vi "create run list.vi"(7 "Group Stanards":string[][](array[string]), 8 "error in (no error)":errorcluster, 9 "Group Unknowns":string[][](array[string]), 10 "Paged groups":string[][][](array[string])=[[["", "", "", "", "", "", ""], ["", "", "", "", "", "", ""], ["", "", "", "", "", "", ""], ["", "", "", "", "", "", ""], ["", "", "", "", "", "", ""], ["", "", "", "", "", "", ""], ["", "", "", "", "", "", ""], ["", "", "", "", "", "", ""], ["", "", "", "", "", "", ""], ["", "", "", "", "", "", ""], ["", "", "", "", "", "", ""], ["", "", "", "", "", "", ""], ["", "", "", "", "", "", ""], ["", "", "", "", "", "", ""]], [["1", "113250", "Owen", "JDP1", "u", "1000", "1"], ["2", "113251", "Owen", "JDP2", "u", "1000", "1"], ["3", "113252", "Owen", "JDP3", "u", "1000", "1"], ["4", "113253", "Owen", "JDP4", "u", "1000", "1"], ["5", "113254", "Owen", "JB1", "u", "1000", "1"], ["6", "113255", "Owen", "JB2", "u", "1000", "1"], ["7", "113256", "Owen", "JB3", "u", "1000", "1"], ["8", "113257", "Owen", "JAC1", "u", "1000", "1"], ["9", "113258", "Owen", "BLK 4", "u", "1000", "1"], ["10", "113259", "Arboleya", "E1", "u", "1000", "1"], ["51", "110511", "Caffee", "KN std Be 0162", "u", "533", "1"], ["52", "110824", "Chmiel", "Blank", "b", "5", "1"], ["55", "96431", "Caffee", "Be-01-5-3 standard", "s", "6320", "1"], ["56", "96432", "Caffee", "Be-01-5-3 standard", "s", "6320", "1"]], [["11", "113260", "Arboleya", "E3", "u", "1000", "2"], ["12", "113261", "Arboleya", "E4", "u", "1000", "2"], ["13", "113262", "Arboleya", "E5", "u", "1000", "2"], ["14", "113263", "Arboleya", "E6", "u", "1000", "2"], ["15", "113264", "Arboleya", "E7", "u", "1000", "2"], ["16", "113265", "Arboleya", "E8", "u", "1000", "2"], ["17", "113266", "Arboleya", "E9", "u", "1000", "2"], ["18", "113267", "Arboleya", "MAR7", "u", "1000", "2"], ["19", "113268", "Arboleya", "BLK7", "u", "1000", "2"], ["20", "113269", "Marshall", "CR101", "u", "1000", "2"], ["57", "96433", "Caffee", "Be-01-5-3 standard", "s", "6320", "2"], ["58", "96434", "Caffee", "Be-01-5-3 standard", "s", "6320", "2"], ["", "", "", "", "", "", ""], ["", "", "", "", "", "", ""]], [["21", "113270", "Marshall", "CR102", "u", "1000", "3"], ["22", "113271", "Marshall", "CR103", "u", "1000", "3"], ["23", "113272", "Marshall", "CR104", "u", "1000", "3"], ["24", "113273", "Marshall", "CR106", "u", "1000", "3"], ["25", "113274", "Marshall", "CR107", "u", "1000", "3"], ["26", "113275", "Marshall", "CR109", "u", "1000", "3"], ["27", "113276", "Marshall", "CR110", "u", "1000", "3"], ["28", "113277", "Marshall", "CR111", "u", "1000", "3"], ["29", "113278", "Marshall", "CR116", "u", "1000", "3"], ["30", "113279", "Marshall", "BLK1", "u", "1000", "3"], ["31", "113280", "Marshall", "CR113", "u", "1000", "3"], ["59", "96435", "Caffee", "Be-01-5-3 standard", "s", "6320", "3"], ["60", "96436", "Caffee", "Be-01-5-3 standard", "s", "6320", "3"], ["", "", "", "", "", "", ""]], [["32", "113281", "Marshall", "CR121", "u", "1000", "4"], ["33", "113282", "Marshall", "CR122", "u", "1000", "4"], ["34", "113283", "Belmont", "W10Vi23I", "u", "1000", "4"], ["35", "113284", "Belmont", "S10X07B", "u", "1000", "4"], ["36", "113285", "Belmont", "S10X08A", "u", "1000", "4"], ["37", "113286", "Belmont", "S10X08B", "u", "1000", "4"], ["38", "113287", "Belmont", "S10X08C", "u", "1000", "4"], ["39", "113288", "Belmont", "S10X08D", "u", "1000", "4"], ["40", "113289", "Belmont", "S10X08E", "u", "1000", "4"], ["41", "113290", "Belmont", "S10X08F", "u", "1000", "4"], ["61", "96437", "Caffee", "Be-01-5-3 standard", "s", "6320", "4"], ["62", "96438", "Caffee", "Be-01-5-3 standard", "s", "6320", "4"], ["", "", "", "", "", "", ""], ["", "", "", "", "", "", ""]], [["42", "113291", "Belmont", "S10X08G", "u", "1000", "5"], ["43", "113292", "Belmont", "Cblk-2560-7", "u", "1000", "5"], ["44", "113293", "Belmont", "S10X08H", "u", "1000", "5"], ["45", "113294", "Belmont", "S10X08I", "u", "1000", "5"], ["46", "113295", "Belmont", "S10X08J", "u", "1000", "5"], ["47", "113296", "Belmont", "S10X08K", "u", "1000", "5"], ["48", "113297", "Belmont", "S10X08L", "u", "1000", "5"], ["49", "113298", "Belmont", "S10X09A", "u", "1000", "5"], ["50", "113299", "Belmont", "S10X09B", "u", "1000", "5"], ["54", "96430", "Caffee", "Be-01-5-3 standard", "s", "6320", "5"], ["63", "96439", "Caffee", "Be-01-5-3 standard", "s", "6320", "5"], ["", "", "", "", "", "", ""], ["", "", "", "", "", "", ""], ["", "", "", "", "", "", ""]], [["", "", "", "", "", "", ""], ["", "", "", "", "", "", ""], ["", "", "", "", "", "", ""], ["", "", "", "", "", "", ""], ["", "", "", "", "", "", ""], ["", "", "", "", "", "", ""], ["", "", "", "", "", "", ""], ["", "", "", "", "", "", ""], ["", "", "", "", "", "", ""], ["", "", "", "", "", "", ""], ["", "", "", "", "", "", ""], ["", "", "", "", "", "", ""], ["", "", "", "", "", "", ""], ["", "", "", "", "", "", ""]], [["", "", "", "", "", "", ""], ["", "", "", "", "", "", ""], ["", "", "", "", "", "", ""], ["", "", "", "", "", "", ""], ["", "", "", "", "", "", ""], ["", "", "", "", "", "", ""], ["", "", "", "", "", "", ""], ["", "", "", "", "", "", ""], ["", "", "", "", "", "", ""], ["", "", "", "", "", "", ""], ["", "", "", "", "", "", ""], ["", "", "", "", "", "", ""], ["", "", "", "", "", "", ""], ["", "", "", "", "", "", ""]]], 11 "number of samples between standards":i32=4 min=1 max=50) -> (0 "error out":errorcluster, 3 "Group run list":string[][](array[string]))   [LabVIEW 2016]
doc: "This vi takes the standard and unknown list data for a group and parses it into a run order"
panel:
  in  "number of times measured":i32=2
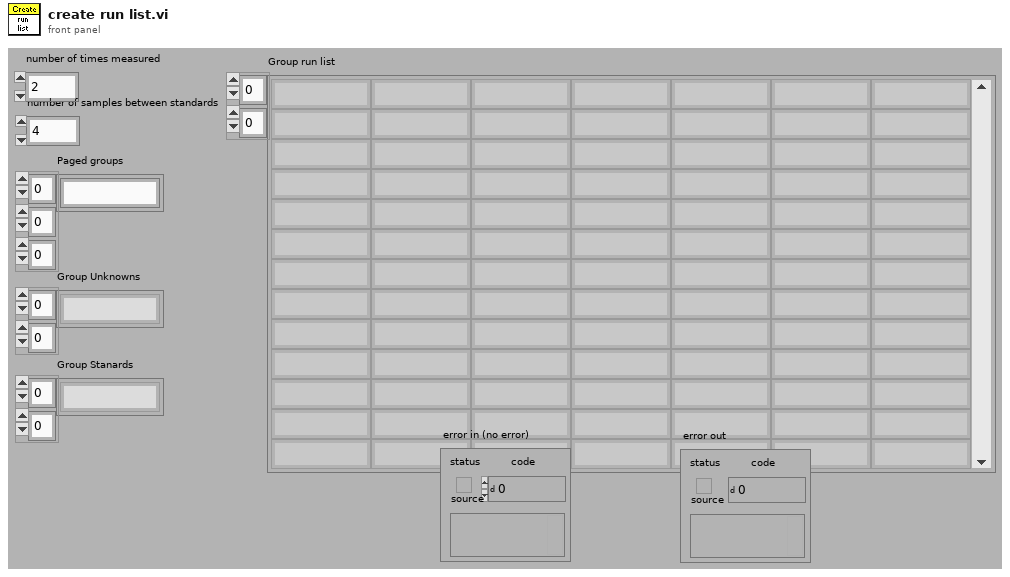
[diagram p1: front panel]
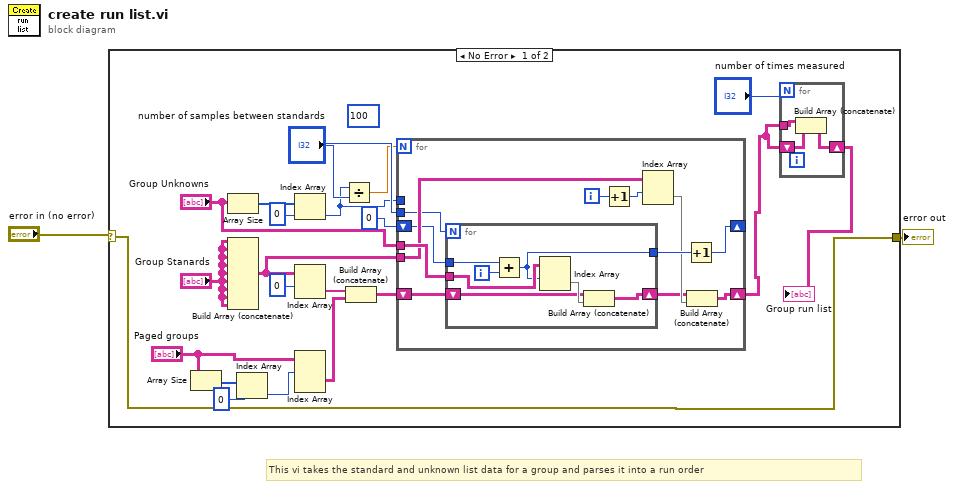
[diagram p0: block diagram]
diagram:
  # "This vi takes the standard and unknown list data for a group and parses it into a run order"
  n1 = case shown="No Error" "error in (no error)" {
    selector: "error in (no error)" -> [w11 w46]
    tunnel: [w11 w46] -> w1
    frame No Error {
      (unwired) 100
      n2 = Array Size(array="Paged groups") -> (size(s)=w9:i32[])
      n3 = Array Size(array="Group Unknowns") -> (size(s)=w13:i32[])
      n4 = Build Array (concatenate)("Group Stanards", "Group Stanards", "Group Stanards", "Group Stanards", "Group Stanards", "Group Stanards", "Group Stanards", "Group Stanards", "Group Stanards") -> (w18:string[][])
      n5 = Index Array(array=w9, index=0) -> (element=w7:i32)
      n6 = Index Array(array=w13, index=0) -> (element=w16:i32)
      n7 = Index Array(array=w18, index (row)=0) -> (element=w20:string[])  [unwired: 1 in]
      n8 = Index Array(array="Paged groups", index (dim 0)=w7) -> (element=w17:string[][])  [unwired: 2 in]
      n9 = Divide(x=w16, y="number of samples between standards") -> (x/y=w6:dbl)
      n10 = Build Array (concatenate)(w20, w17) -> (w21:string[][])
      n11 = for {
        N: w6 -> [_]
        tunnel: w16 -> [_]
        tunnel: "Group Unknowns" -> [w38]
        tunnel: w18 -> [w35]
        shift-right: [w27] -> w3
        shift-left: w21 -> [w30]
        tunnel: "number of samples between standards" -> [w34]
        shift-right: [w32] -> _
        shift-left: 0 ("index") -> [w31]
        i -> [w37]
        n12 = for {
          N: w34 -> [_]
          tunnel: w38 -> [w43]
          tunnel: w31 -> [w44]
          tunnel: [w42] -> w33
          shift-right: [w40] -> w28
          shift-left: w30 -> [w39]
          i -> [w45]
          n13 = Add(x=w44, y=w45) -> (x+y=w42:i32)
          n14 = Index Array(array=w43, index (row)=w42) -> (element=w41:string[])  [unwired: 1 in]
          n15 = Build Array (concatenate)(w39, w41) -> (w40:string[][])
        }
        n16 = Increment(x=w37) -> (x+1=w36:i32)
        n17 = Index Array(array=w35, index (row)=w36) -> (element=w29:string[])  [unwired: 1 in]
        n18 = Increment(x=w33) -> (x+1=w32:i32)
        n19 = Build Array (concatenate)(w28, w29) -> (w27:string[][])
      }
      n20 = for {
        N: "number of times measured" -> [_]
        shift-right: [w26] -> w4
        shift-left: w3 -> [w25]
        tunnel: w3 -> [w24]
        n21 = Build Array (concatenate)(w24, w25) -> (w26:string[][])
      }
      "Group run list" <- w4
    }
    frame Error {
    }
  }
  "error out" <- w1
